vi "Read SA Pin.vi"(8 "error in (no error)":errorcluster, 11 "Skyworks - PVT in":refnum<class "Skyworks - PVT.lvclass">) -> (0 "error out":errorcluster, 2 "SA Pin":string, 3 "Skyworks - PVT out":refnum<class "Skyworks - PVT.lvclass">)   [LabVIEW 2018, in "Skyworks PVT.lvlib" / "Skyworks - PVT.lvclass"]
uses:
  Skyworks - PVT.lvclass
  Skyworks - PVT.lvclass/Skyworks - PVT.ctl
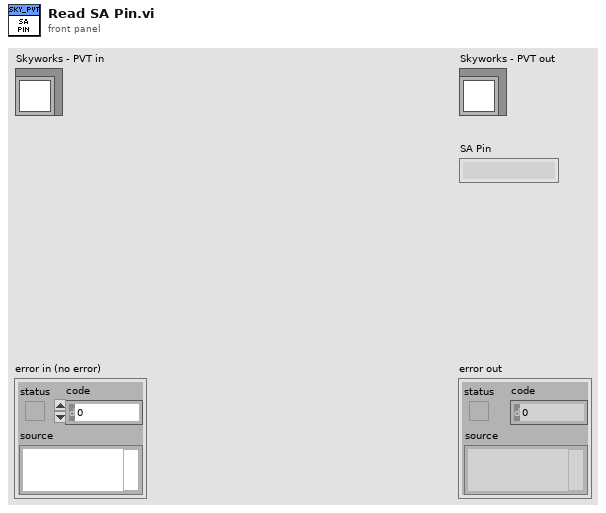
[diagram p1: front panel]
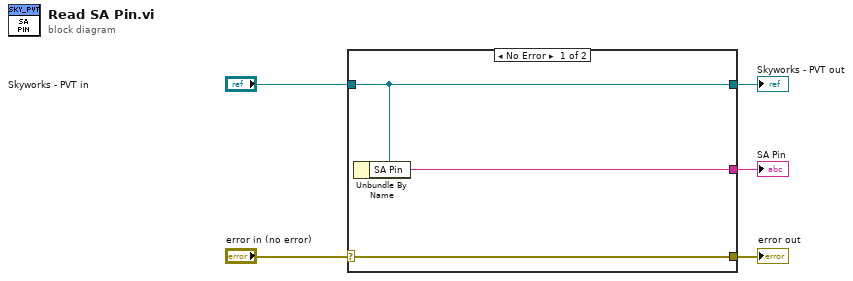
[diagram p0: block diagram]
diagram:
  n1 = case shown="No Error" "error in (no error)" {
    selector: "error in (no error)" -> [w8 w9]
    tunnel: [w8 w9] -> w4
    tunnel: [w7 w10] -> w2
    tunnel: "Skyworks - PVT in" -> [w7 w10]
    tunnel: [w6 _] -> w1
    frame No Error {
      n2 = Unbundle By Name(w7) -> ("SA Pin"=w6:string)
    }
    frame Error {
    }
  }
  "error out" <- w4
  "Skyworks - PVT out" <- w2
  "SA Pin" <- w1
